vi "2023 Test Arm To Phi Logic.vi"() -> ()   [LabVIEW 2020]
panel:
  out "y value":dbl
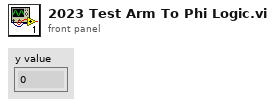
[diagram p1: front panel]
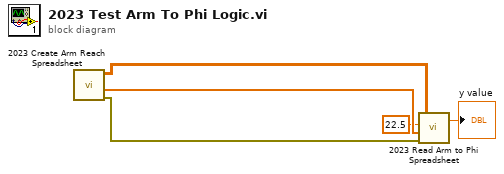
[diagram p0: block diagram]
diagram:
  n1 = call "2023 Create Arm Reach Spreadsheet.vi"() -> ("transposed array"=w4:dbl[][], "output array 2"=w3:dbl[], "error out"=w5:errorcluster)  [unwired: 1 in, 1 out]
  n2 = call "2023 Read Arm to Phi Spreadsheet.vi"("error in"=w5, "output array 2"=w3, "Arm Angle"=22.5, "transposed array"=w4) -> ("y value"=→"y value":dbl)  [unwired: 1 out]
